vi "Encoder globals.vi"() -> ()   [LabVIEW 2013]
panel:
  out "Encoder Error":errorcluster
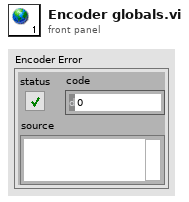
[diagram p1: front panel]
diagram:
